vi "parse load from file.vi"(8 "error in":errorcluster, 11 "message data":string) -> (0 "error out":errorcluster, 2 "target alias":string, 3 "path":path)   [LabVIEW 2013, in "DCAF Execution Service.lvlib"]
uses:
  DCAF Execution Service.lvlib
  tokenized path.ctl
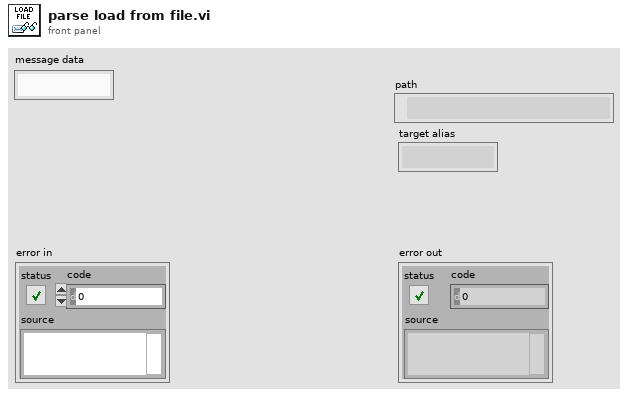
[diagram p1: front panel]
types:
  T1 = typedef "DCAF Execution Service.lvlib/tokenized path.ctl" = string[]
  T2 = cluster{"tokenized path":T1, "target alias":string}
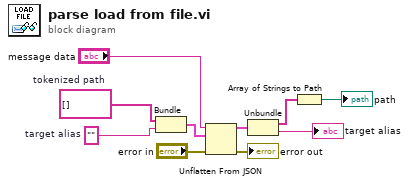
[diagram p0: block diagram]
diagram:
  w2 = ""  # target alias
  w3 = T1 []  # tokenized path
  n1 = Bundle("tokenized path"=w3, "target alias"=w2) -> (w7:T2)  [unwired: 1 in]
  n2 = Unflatten From JSON(JSON string="message data", type and defaults=w7, error in (no error)="error in") -> (value=w6:T2, error out=→"error out":errorcluster)  [unwired: 4 in]
  n3 = Unbundle(w6) -> ("tokenized path"=w5:T1, "target alias"=→"target alias":string)
  n4 = Array of Strings to Path(0:w5) -> (2:→"path":path)  [unwired: 1 in]
